vi "Periodic Tasks.vi"(8 "error in":errorcluster) -> ()   [LabVIEW 2017]
doc: "This VI runs in parallel to other tasks. It can contain as many user-defined periodic loops as you need. These can carry out PID or other sorts of timed response."
uses:
  <vilib>/Rock Robotics/WPI/DriverStation/WPI_DriverStationRobotMode2.ctl
  <vilib>/Rock Robotics/WPI/ThirdParty/Phoenix-LabVIEW/Motor Controller/Controls/CTRE_Phoenix_MotorControl_ControlMode.ctl
  <vilib>/Rock Robotics/WPI/Utilities/WPI_GetSetVariantRefNum.vi
  Robot Global Data.vi
  <vilib>/Rock Robotics/Network Tables/NT Write String.vi
  <vilib>/Rock Robotics/WPI/ThirdParty/Phoenix-LabVIEW/Motor Controller/Get/CTRE_Phoenix_MotorController_GetPulseWidthAll.vi
  <vilib>/Rock Robotics/Network Tables/NT Write Number.vi
  <vilib>/Rock Robotics/WPI/ThirdParty/Phoenix-LabVIEW/Motor Controller/Get/CTRE_Phoenix_MotorController_GetQuadratureData.vi
  <vilib>/Rock Robotics/Network Tables/NT Write Numeric Array.vi
  <vilib>/Rock Robotics/WPI/Solenoid/WPI_SolenoidGetEnum.vi
  <vilib>/Rock Robotics/WPI/RobotDrive/WPI_RobotDriveArcadeDrive_Standard(NoSaturation).vi
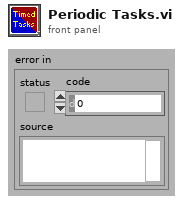
[diagram p1: front panel]
types:
  T1 = typedef "WPI_CompressorDevRef.ctl" = cluster{"DevStatus":errorcluster, "Pneumatics Control Module":u8}
  T2 = typedef "WPI_JoystickDevRef.ctl" = cluster{"Device":T3}
  T3 = typedef "WPI_JoystickDeviceEnum.ctl" = enum16{"USB 0", "USB 1", "USB 2", "USB 3", "USB 4", "USB 5"}
  T4 = typedef "WPI_MotorControlDeviceRef.ctl" = cluster{"DeviceStatus":errorcluster, "Type":T5, "PWM":cluster{"PWM Channel":T6, "DeadBand":T7}, "CAN":cluster{"Device Number":u8, "SetOutput VI Ref":variant, "GetOutput VI Ref":variant, "Enable VI Ref":variant, "Disable VI Ref":variant, "Data":variant}, "Invert":bool, "DIO PWM":cluster{"PWM \"Enable\" Channel":T6, "DIOChannel":T8, "PWM Rate":dbl}}
  T5 = typedef "WPI_MotorControlType.ctl" = enum16{"PWM", "CAN", "DIO PWM"}
  T6 = typedef "FPGA_DIOPWMChannel.ctl" = enum8{"PWM 0", "PWM 1", "PWM 2", "PWM 3", "PWM 4", "PWM 5", "PWM 6", "PWM 7", "PWM 8", "PWM 9", "PWM MXP 0", "PWM MXP 1", "PWM MXP 2", "PWM MXP 3", "PWM MXP 4", "PWM MXP 5", "PWM MXP 6", "PWM MXP 7", "PWM MXP 8", "PWM MXP 9", "Invalid"}
  T7 = typedef "WPI_PWMDeadband.ctl" = cluster{"Name":string, "maxPositivePwm":i32, "minPositivePwm":i32, "centerPwm":i32, "maxNegativePwm":i32, "minNegativePwm":i32, "angularRange":u16}
  T8 = typedef "FPGA_DIOChannel.ctl" = enum8{"DIO 0", "DIO 1", "DIO 2", "DIO 3", "DIO 4", "DIO 5", "DIO 6", "DIO 7", "DIO 8", "DIO 9", "DIO MXP 0", "DIO MXP 1", "DIO MXP 2", "DIO MXP 3", "DIO MXP 4", "DIO MXP 5", "DIO MXP 6", "DIO MXP 7", "DIO MXP 8", "DIO MXP 9", "DIO MXP 10", "DIO MXP 11", "DIO MXP 12", "DIO MXP 13", "DIO MXP 14", "DIO MXP 15", "SPI Port CS1", "SPI Port CS2", "SPI Port CS3", "SPI Port MISO", "SPI Port MOSI", "Invalid"}
  T9 = typedef "WPI_SolenoidDevRef.ctl" = cluster{"DevStatus":errorcluster, "Pneumatics Control Module":u8, "Forward Solenoid Channel":T10, "Reverse Solenoid Channel":T10}
  T10 = typedef "WPI_SolenoidChannel.ctl" = enum8{"Solenoid 0", "Solenoid 1", "Solenoid 2", "Solenoid 3", "Solenoid 4", "Solenoid 5", "Solenoid 6", "Solenoid 7", "Invalid"}
  T11 = typedef "WPI_GyroDevRef.ctl" = cluster{"DevStatus":errorcluster, "Analog Channel":T12, "Gain (VoltsPerDegree/Second)":dbl, "Gyro Type":enum16{"Analog", "XRS450"}, "Handle":i32, "SPI Bus":T13, "Device Found":bool, "Sample Rate":dbl, "Calibrate On Open":bool, "Offset":dbl}
  T12 = typedef "FPGA_AIChannel.ctl" = enum8{"AI 0", "AI 1", "AI 2", "AI 3", "AI MXP 0", "AI MXP 1", "AI MXP 2", "AI MXP 3", "Invalid"}
  T13 = typedef "spi_bus.ctl" = enum16{"SPI On-Board, CS0", "SPI On-Board, CS1", "SPI On-Board, CS2", "SPI On-Board, CS3", "SPI MXP", "Invalid"}
  T14 = typedef "WPI_RobotDriveDevRef.ctl" = cluster{"DevStatus":errorcluster, "Motors[]":T4[], "Square Inputs":bool, "Max Output":dbl}
  T15 = cluster{"GyroDevRef":T11, "JoystickDevRef":T2, "RobotDriveDevRef":T14, "PhoenixMotorControlDevRef":T4, "PhoenixMotorControlDevRef":T4, "PhoenixMotorControlDevRef":T4, "PhoenixMotorControlDevRef":T4, "PhoenixMotorControlDevRef":T4, "PhoenixMotorControlDevRef":T4, "SolenoidDevRef":T9}
  T16 = typedef "WPI_DriverStationRobotMode2.ctl" = enum16{"Autonomous Disabled", "Autonomous Enabled", "Teleop Disabled", "Teleop Enabled", "Disconnected", "Finish", "Test Disabled", "Test Enabled", "Emergency Stopped"}
  T17 = typedef "WPI_SolenoidValue.ctl" = enum16{"Off", "On", "Forward", "Reverse"}
  T18 = enum16{"Arm Down", "Arm Switch", "Arm(Low Scale)", "Arm(Normal Scale)", "Arm(High Scale)", "Hang"}
  T19 = typedef "CTRE_Phoenix_MotorControl_ControlMode.ctl" = u16
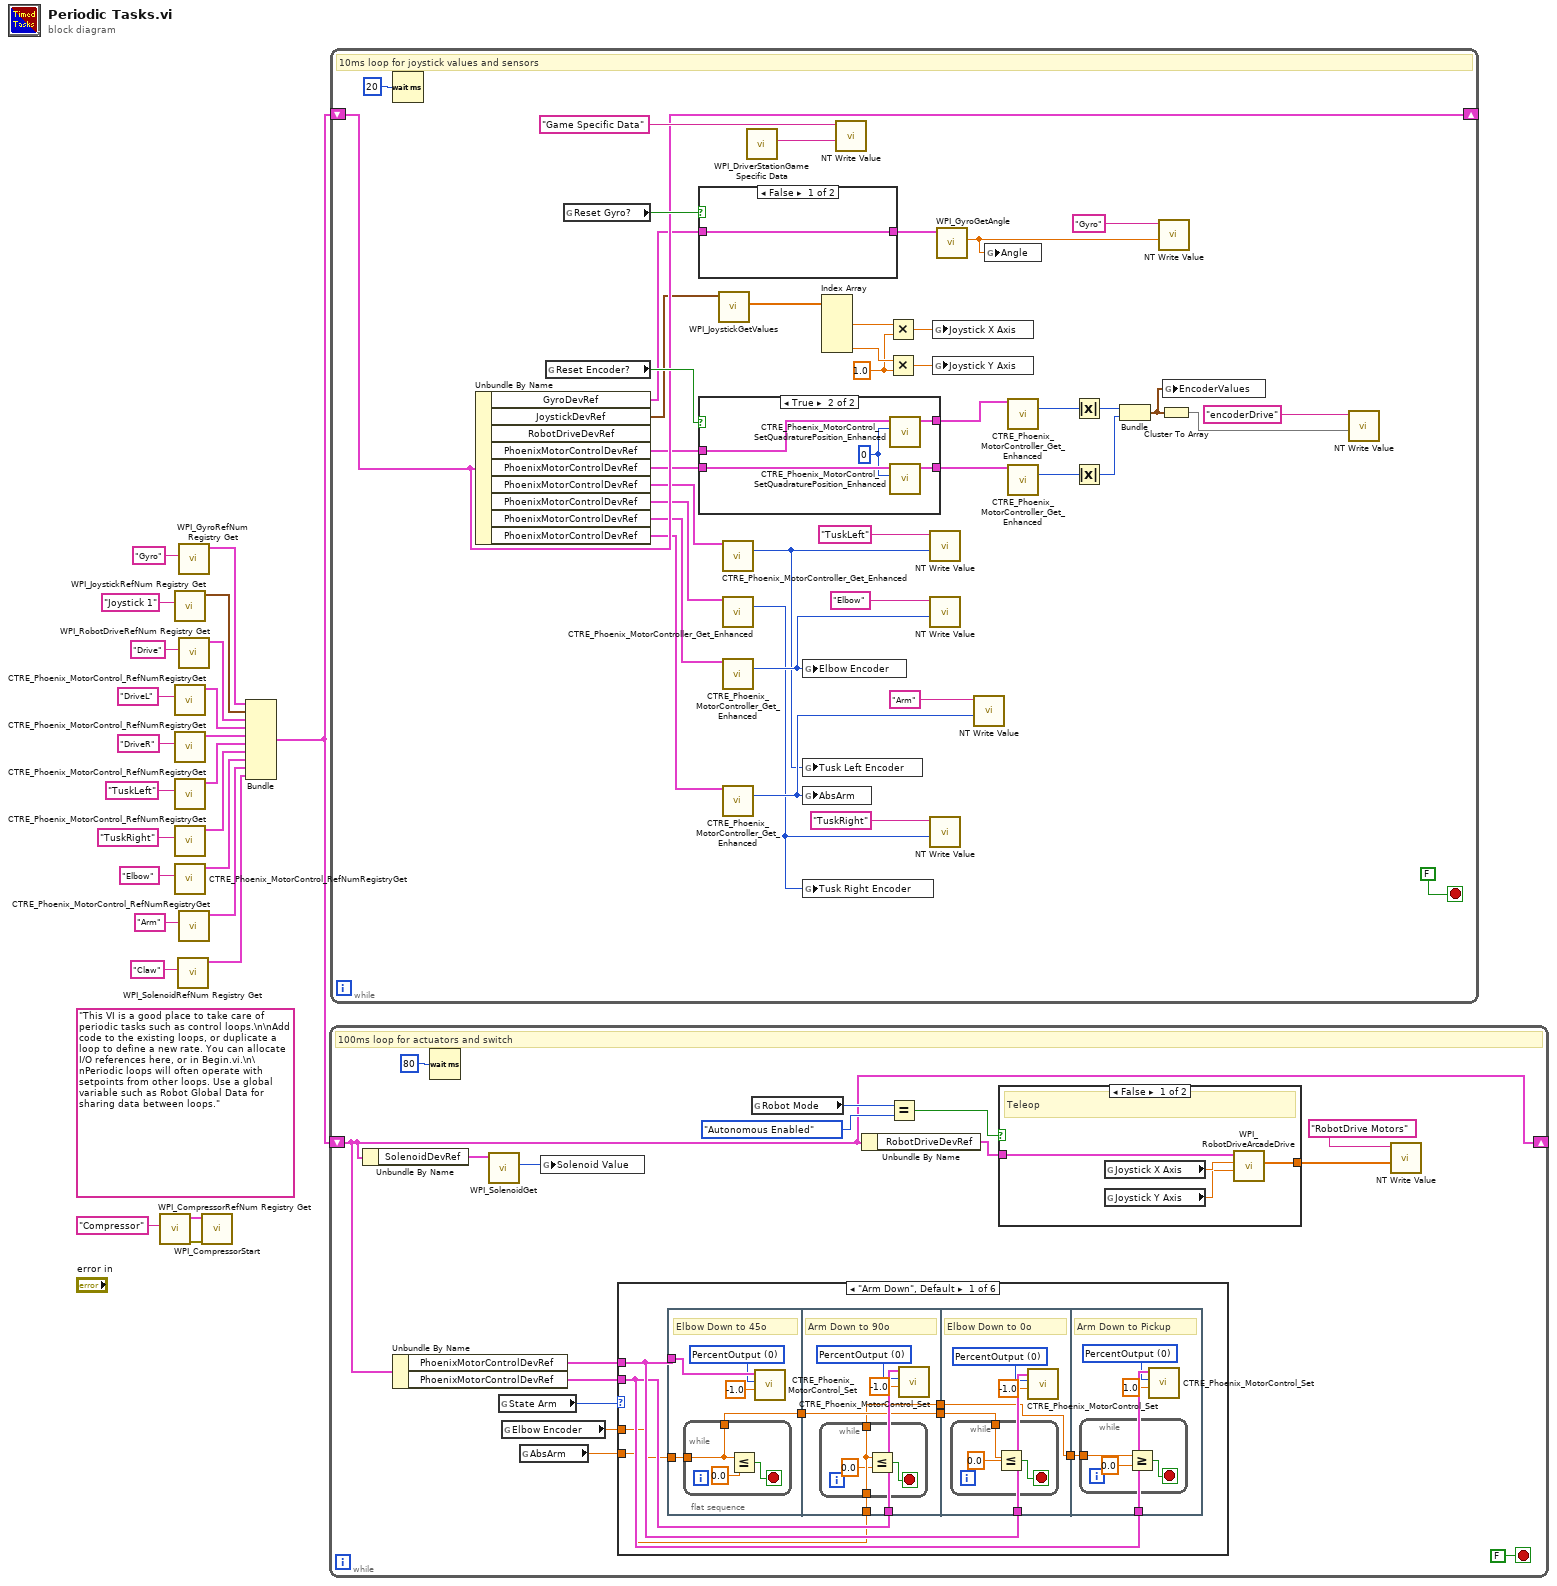
[diagram p0: block diagram]
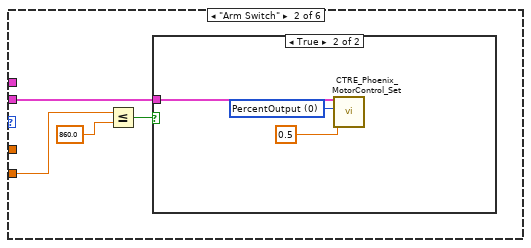
[diagram p2: hidden frame]
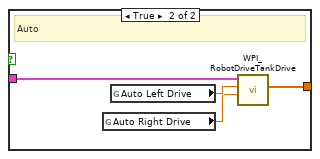
[diagram p8: hidden frame]
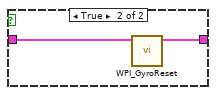
[diagram p9: hidden frame]
diagram:
  (unwired) "This VI is a good place to take care of periodic tasks such as control loops.\n\nAdd code to the existing loops, or duplicate a loop to define a new rate. You can allocate I/O references here, or in Begin.vi.\n\nPeriodic loops will often operate with setpoints from other loops. Use a global variable such as Robot Global Data for sharing data between loops."
  n1 = call <vilib>:"WPI_CompressorRefNum Registry Get.vi"("refnum name"="Compressor") -> ("error out"=w20:errorcluster, "CompressorDevRef"=w19:T1)  [unwired: 9 in]
  n2 = call <vilib>:"WPI_JoystickRefNum Registry Get.vi"("refnum name"="Joystick 1") -> ("JoystickDevRef"=w10:T2)  [unwired: 1 in, 9 out]
  n3 = call <vilib>:"CTRE_Phoenix_MotorControl_RefNumRegistryGet.vi"("refnum name"="DriveL") -> ("PhoenixMotorControlDevRef"=w8:T4)  [unwired: 9 in, 1 out]
  n4 = call <vilib>:"CTRE_Phoenix_MotorControl_RefNumRegistryGet.vi"("refnum name"="DriveR") -> ("PhoenixMotorControlDevRef"=w7:T4)  [unwired: 9 in, 1 out]
  n5 = call <vilib>:"CTRE_Phoenix_MotorControl_RefNumRegistryGet.vi"("refnum name"="TuskLeft") -> ("PhoenixMotorControlDevRef"=w6:T4)  [unwired: 9 in, 1 out]
  n6 = call <vilib>:"CTRE_Phoenix_MotorControl_RefNumRegistryGet.vi"("refnum name"="TuskRight") -> ("PhoenixMotorControlDevRef"=w5:T4)  [unwired: 9 in, 1 out]
  n7 = call <vilib>:"CTRE_Phoenix_MotorControl_RefNumRegistryGet.vi"("refnum name"="Elbow") -> ("PhoenixMotorControlDevRef"=w4:T4)  [unwired: 9 in, 1 out]
  n8 = call <vilib>:"WPI_SolenoidRefNum Registry Get.vi"("refnum name"="Claw") -> ("SolenoidDevRef"=w2:T9)  [unwired: 9 in, 1 out]
  n9 = call <vilib>:"WPI_GyroRefNum Registry Get.vi"("refnum name"="Gyro") -> ("GyroDevRef"=w11:T11)  [unwired: 9 in, 1 out]
  n10 = call <vilib>:"WPI_RobotDriveRefNum Registry Get.vi"("refnum name"="Drive") -> ("RobotDriveDevRef"=w9:T14)  [unwired: 1 in, 9 out]
  n11 = call <vilib>:"CTRE_Phoenix_MotorControl_RefNumRegistryGet.vi"("refnum name"="Arm") -> ("PhoenixMotorControlDevRef"=w3:T4)  [unwired: 9 in, 1 out]
  n12 = call <vilib>:"WPI_CompressorStart.vi"("error in (no error)"=w20, "CompressorDevRef"=w19) -> ()  [unwired: 8 in, 2 out]
  n13 = Bundle("GyroDevRef"=w11, "JoystickDevRef"=w10, "RobotDriveDevRef"=w9, "PhoenixMotorControlDevRef"=w8, "PhoenixMotorControlDevRef"=w7, "PhoenixMotorControlDevRef"=w6, "PhoenixMotorControlDevRef"=w5, "PhoenixMotorControlDevRef"=w4, "PhoenixMotorControlDevRef"=w3, "SolenoidDevRef"=w2) -> (w1:T15)  [unwired: 1 in]
  n14 = while {
    shift-right: [w29] -> _
    shift-left: w1 -> [w29]
    stop <- FALSE stop-if-true
    # "100ms loop for actuators and switch"
    n15 = Unbundle By Name(w29) -> ("SolenoidDevRef"=w32:T9)
    n16 = Unbundle By Name(w29) -> ("PhoenixMotorControlDevRef"=w27:T4, "PhoenixMotorControlDevRef"=w28:T4)
    n17 = Wait (ms)(milliseconds to wait=u32 80) -> ()  [unwired: 1 out]
    n18 = call-poly <vilib>:"WPI_SolenoidGet.vi"("SolenoidDevRef"=w32) -> ("Value"=w31:T17)  [unwired: 8 in, 2 out]
    n19 = global read "Robot Global Data.vi" "State Arm"() -> (w30:T18)
    n20 = global read "Robot Global Data.vi" "Elbow Encoder"() -> (w26:dbl)
    n21 = global read "Robot Global Data.vi" "AbsArm"() -> (w25:dbl)
    n22 = global write "Robot Global Data.vi" "Solenoid Value"(w31) -> ()
    n23 = case shown="\"Arm Down\", Default" w30 {
      tunnel: w28 -> [w47 w81 _ _ _ _]
      tunnel: w27 -> [w48 _ _ _ _ _]
      tunnel: w26 -> [w46 _ _ _ _ _]
      tunnel: w25 -> [w45 w84 _ _ _ _]
      frame "Arm Down", Default {
        n24 = flat-sequence {
          tunnel: w48 -> [w53]
          tunnel: w46 -> [w51]
          tunnel: [w50] -> w43
          tunnel: w47 -> [w62]
          tunnel: w45 -> [w60]
          tunnel: [w59] -> w44
          tunnel: w43 -> [w59]
          tunnel: [w58] -> w41
          tunnel: w48 -> [w70]
          tunnel: w44 -> [w68]
          tunnel: [w67] -> w42
          tunnel: w41 -> [w67]
          tunnel: w47 -> [w77]
          tunnel: w42 -> [w75]
          frame #0 {
            w52 = T19 0 items=["PercentOutput"=0, "Position"=1, "Velocity"=2, "Current"=3, "Follower"=5, "MotionProfile"=6, "MotionMagic"=7, "MotionMagicArc"=8, "MotionProfileArc"=10, "Disabled"=15] ("Control Mode")
            # "Elbow Down to 45o"
            n25 = while {
              tunnel: w51 -> [w55]
              tunnel: [w55] -> w50
              stop <- w56 stop-if-true
              n26 = Less Or Equal?(x=w55, y=0.0) -> (x <= y?=w56:bool)
            }
            n27 = call <vilib>:"CTRE_Phoenix_MotorControl_Set.vi"("Output"=-1.0, "Control Mode"=w52, "PhoenixMotorControlDevRef"=w53) -> ()  [unwired: 7 in, 2 out]
          }
          frame #1 {
            w61 = T19 0 items=["PercentOutput"=0, "Position"=1, "Velocity"=2, "Current"=3, "Follower"=5, "MotionProfile"=6, "MotionMagic"=7, "MotionMagicArc"=8, "MotionProfileArc"=10, "Disabled"=15] ("Control Mode")
            # "Arm Down to 90o"
            n28 = while {
              tunnel: w60 -> [w64]
              tunnel: [w64] -> w58
              stop <- w65 stop-if-true
              n29 = Less Or Equal?(x=w64, y=0.0) -> (x <= y?=w65:bool)
            }
            n30 = call <vilib>:"CTRE_Phoenix_MotorControl_Set.vi"("Output"=-1.0, "Control Mode"=w61, "PhoenixMotorControlDevRef"=w62) -> ()  [unwired: 7 in, 2 out]
          }
          frame #2 {
            w69 = T19 0 items=["PercentOutput"=0, "Position"=1, "Velocity"=2, "Current"=3, "Follower"=5, "MotionProfile"=6, "MotionMagic"=7, "MotionMagicArc"=8, "MotionProfileArc"=10, "Disabled"=15] ("Control Mode")
            # "Elbow Down to 0o"
            n31 = while {
              tunnel: w68 -> [w72]
              stop <- w73 stop-if-true
              n32 = Less Or Equal?(x=w72, y=0.0) -> (x <= y?=w73:bool)
            }
            n33 = call <vilib>:"CTRE_Phoenix_MotorControl_Set.vi"("Output"=-1.0, "Control Mode"=w69, "PhoenixMotorControlDevRef"=w70) -> ()  [unwired: 7 in, 2 out]
          }
          frame #3 {
            w76 = T19 0 items=["PercentOutput"=0, "Position"=1, "Velocity"=2, "Current"=3, "Follower"=5, "MotionProfile"=6, "MotionMagic"=7, "MotionMagicArc"=8, "MotionProfileArc"=10, "Disabled"=15] ("Control Mode")
            # "Arm Down to Pickup"
            n34 = while {
              tunnel: w75 -> [w79]
              stop <- w80 stop-if-true
              n35 = Greater Or Equal?(x=w79, y=0.0) -> (x >= y?=w80:bool)
            }
            n36 = call <vilib>:"CTRE_Phoenix_MotorControl_Set.vi"("Output"=1.0, "Control Mode"=w76, "PhoenixMotorControlDevRef"=w77) -> ()  [unwired: 7 in, 2 out]
          }
        }
      }
      frame "Arm Switch" {
        n37 = Less Or Equal?(x=w84, y=860.0) -> (x <= y?=w82:bool)
        n38 = case shown="True" w82 {
          tunnel: w81 -> [_ w87]
          frame False {
          }
          frame True {
            w86 = T19 0 items=["PercentOutput"=0, "Position"=1, "Velocity"=2, "Current"=3, "Follower"=5, "MotionProfile"=6, "MotionMagic"=7, "MotionMagicArc"=8, "MotionProfileArc"=10, "Disabled"=15] ("Control Mode")
            n39 = call <vilib>:"CTRE_Phoenix_MotorControl_Set.vi"("Output"=0.5, "Control Mode"=w86, "PhoenixMotorControlDevRef"=w87) -> ()  [unwired: 7 in, 2 out]
          }
        }
      }
      frame "Arm(Low Scale)" {
      }
      frame "Arm(Normal Scale)" {
      }
      frame "Arm(High Scale)" {
      }
      frame "Hang" {
      }
    }
    n40 = global read "Robot Global Data.vi" "Robot Mode"() -> (w37:T16)
    n41 = Unbundle By Name(w29) -> ("RobotDriveDevRef"=w35:T14)
    n42 = Equal?(x=w37, y=WPI_DriverStationRobotMode2."Autonomous Enabled") -> (x = y?=w38:bool)
    n43 = case shown="False" w38 {
      tunnel: w35 -> [w91 w92]
      tunnel: [w88 w95] -> w33
      frame False {
        # "Teleop"
        n44 = global read "Robot Global Data.vi" "Joystick X Axis"() -> (w90:dbl)
        n45 = global read "Robot Global Data.vi" "Joystick Y Axis"() -> (w89:dbl)
        n46 = call-poly <vilib>:"WPI_RobotDriveArcadeDrive.vi"("Y axis value"=w89, "X axis value"=w90, "RobotDriveDevRef"=w91) -> ("Motor Values"=w88:dbl[])  [unwired: 6 in, 2 out]
      }
      frame True {
        # "Auto"
        n47 = global read "Robot Global Data.vi" "Auto Right Drive"() -> (w93:dbl)
        n48 = global read "Robot Global Data.vi" "Auto Left Drive"() -> (w94:dbl)
        n49 = call <vilib>:"WPI_RobotDriveTankDrive.vi"("Right axis value"=w93, "Left axis value"=w94, "RobotDriveDevRef"=w92) -> ("Motor Values"=w95:dbl[])  [unwired: 6 in, 2 out]
      }
    }
    n50 = call-poly <vilib>:"NT Write Value.vi"("Numeric Array"=w33, "Name"="RobotDrive Motors") -> ()  [unwired: 9 in, 1 out]
  }
  n51 = while {
    shift-right: [w108] -> _
    shift-left: w1 -> [w108]
    stop <- FALSE stop-if-true
    w129 = 1.0
    # "10ms loop for joystick values and sensors"
    n52 = Wait (ms)(milliseconds to wait=u32 20) -> ()  [unwired: 1 out]
    n53 = Unbundle By Name(w108) -> ("GyroDevRef"=w107:T11, "JoystickDevRef"=w106:T2, "PhoenixMotorControlDevRef"=w105:T4, "PhoenixMotorControlDevRef"=w104:T4, "PhoenixMotorControlDevRef"=w103:T4, "PhoenixMotorControlDevRef"=w102:T4, "PhoenixMotorControlDevRef"=w101:T4, "PhoenixMotorControlDevRef"=w100:T4)  [unwired: 1 out]
    n54 = global read "Robot Global Data.vi" "Reset Encoder?"() -> (w124:bool)
    n55 = global read "Robot Global Data.vi" "Reset Gyro?"() -> (w122:bool)
    n56 = case shown="False" w122 {
      tunnel: w107 -> [w137 w139]
      tunnel: [w137 w138] -> w123
      frame False {
      }
      frame True {
        n57 = call <vilib>:"WPI_GyroReset.vi"("GyroDevRef"=w139) -> ("GyroDevRef"=w138:T11)  [unwired: 9 in, 1 out]
      }
    }
    n58 = case shown="True" w124 {
      tunnel: w105 -> [w141 w146]
      tunnel: w104 -> [w140 w144]
      tunnel: [w141 w145] -> w126
      tunnel: [w140 w143] -> w125
      frame False {
      }
      frame True {
        w142 = 0 ("New Position")
        n59 = call <vilib>:"CTRE_Phoenix_MotorControl_SetQuadraturePosition_Enhanced.vi"("New Position"=w142, "PhoenixMotorControlDevRef"=w146) -> ("PhoenixMotorControlDevRef"=w145:T4)  [unwired: 8 in, 1 out]
        n60 = call <vilib>:"CTRE_Phoenix_MotorControl_SetQuadraturePosition_Enhanced.vi"("New Position"=w142, "PhoenixMotorControlDevRef"=w144) -> ("PhoenixMotorControlDevRef"=w143:T4)  [unwired: 8 in, 1 out]
      }
    }
    n61 = call <vilib>:"WPI_JoystickGetValues.vi"("JoystickDevRef"=w106) -> ("Axes"=w134:dbl[])  [unwired: 6 in, 4 out]
    n62 = call-poly <vilib>:"CTRE_Phoenix_MotorController_Get_Enhanced.vi"("PhoenixMotorControlDevRef"=w103) -> ("Pulse Width Position"=w96:i32)  [unwired: 9 in, 5 out]
    n63 = call-poly <vilib>:"CTRE_Phoenix_MotorController_Get_Enhanced.vi"("PhoenixMotorControlDevRef"=w102) -> ("Pulse Width Position"=w97:i32)  [unwired: 9 in, 5 out]
    n64 = call-poly <vilib>:"CTRE_Phoenix_MotorController_Get_Enhanced.vi"("PhoenixMotorControlDevRef"=w101) -> ("Pulse Width Position"=w98:i32)  [unwired: 9 in, 5 out]
    n65 = call-poly <vilib>:"CTRE_Phoenix_MotorController_Get_Enhanced.vi"("PhoenixMotorControlDevRef"=w100) -> ("Pulse Width Position"=w99:i32)  [unwired: 9 in, 5 out]
    n66 = call <vilib>:"WPI_DriverStationGame Specific Data.vi"() -> ("Game Specific Data"=w117:string)  [unwired: 11 in]
    n67 = global write "Robot Global Data.vi" "Elbow Encoder"(w98) -> ()
    n68 = global write "Robot Global Data.vi" "Tusk Left Encoder"(w96) -> ()
    n69 = global write "Robot Global Data.vi" "AbsArm"(w99) -> ()
    n70 = global write "Robot Global Data.vi" "Tusk Right Encoder"(w97) -> ()
    n71 = Index Array(array=w134) -> (element #2=w131:dbl, element #5=w130:dbl)  [unwired: 5 in, 3 out]
    n72 = call-poly <vilib>:"NT Write Value.vi"("String"=w117, "Name"="Game Specific Data") -> ()  [unwired: 9 in, 1 out]
    n73 = Multiply(x=w131, y=w129) -> (x*y=w132:dbl)
    n74 = Multiply(x=w130, y=w129) -> (x*y=w133:dbl)
    n75 = call-poly <vilib>:"NT Write Value.vi"("Numeric"=w96, "Name"="TuskLeft") -> ()  [unwired: 9 in, 1 out]
    n76 = call-poly <vilib>:"NT Write Value.vi"("Numeric"=w98, "Name"="Elbow") -> ()  [unwired: 9 in, 1 out]
    n77 = call-poly <vilib>:"NT Write Value.vi"("Numeric"=w97, "Name"="TuskRight") -> ()  [unwired: 9 in, 1 out]
    n78 = global write "Robot Global Data.vi" "Joystick X Axis"(w132) -> ()
    n79 = global write "Robot Global Data.vi" "Joystick Y Axis"(w133) -> ()
    n80 = call <vilib>:"WPI_GyroGetAngle.vi"("GyroDevRef"=w123) -> ("Angle"=w128:dbl)  [unwired: 6 in, 4 out]
    n81 = call-poly <vilib>:"NT Write Value.vi"("Numeric"=w99, "Name"="Arm") -> ()  [unwired: 9 in, 1 out]
    n82 = global write "Robot Global Data.vi" "Angle"(w128) -> ()
    n83 = call-poly <vilib>:"CTRE_Phoenix_MotorController_Get_Enhanced.vi"("PhoenixMotorControlDevRef"=w126) -> ("Quadrature Position"=w118:i32)  [unwired: 11 in, 3 out]
    n84 = call-poly <vilib>:"CTRE_Phoenix_MotorController_Get_Enhanced.vi"("PhoenixMotorControlDevRef"=w125) -> ("Quadrature Position"=w121:i32)  [unwired: 11 in, 3 out]
    n85 = Absolute Value(x=w118) -> (abs(x)=w119:i32)
    n86 = Absolute Value(x=w121) -> (abs(x)=w120:i32)
    n87 = Bundle(w119, w120) -> (w110:cluster{i32, i32})  [unwired: 1 in]
    n88 = call-poly <vilib>:"NT Write Value.vi"("Numeric"=w128, "Name"="Gyro") -> ()  [unwired: 9 in, 1 out]
    n89 = Cluster To Array(cluster=w110) -> (array=w109:i32[])
    n90 = global write "Robot Global Data.vi" "EncoderValues"(w110) -> ()
    n91 = call-poly <vilib>:"NT Write Value.vi"("Numeric Array"=w109, "Name"="encoderDrive") -> ()  [unwired: 9 in, 1 out]
  }
